vi "labHolo2.vi"() -> ()   [LabVIEW 2022 SP3]
uses:
  <vilib>/Analysis/NI_AALBase.lvlib
panel:
  in  "Mod. func.":string
  in  "SLM calibration":u16(ring) items=["211209_lowFreq", "a20220523", "IDSfirst"]
  in  "Reset reff.":bool
  in  "RefTimeSeries 2":dbl[](array[numeric])=array[4424 elements]
  out "Reff alert":bool
  out "size":i32=378225
  out "Reff ROI":T1={"Global Rectangle"=[2653, 1459, 3268, 2074], "Contours"=[{"Contour Type"=0, "ROI Type"=3, "Points"=[2653, 1459, 3268, 2074]}]}
  in  "RefTimeSeries":dbl[](array[numeric])=array[4424 elements]
  in  "take reff":bool
  out "ROI":T1={"Global Rectangle"=[437, 929, 1461, 1953], "Contours"=[{"Contour Type"=0, "ROI Type"=3, "Points"=[437, 929, 1461, 1953]}]}
  in  "Auto. hist":bool caption="Auto."
  out "ROI size":i32=1048576
  out "mean":dbl=2640.427523612976
  out "mean bar":dbl(slide)=2640.427523612976 scale=0.0..200.0
  in  "Whole/ROI":bool=TRUE
  out "max":i16=4095
  out "Histograph":T2(graph)={"Starting Value"=0.0, "Incremental Value"=1.0002441, "Histogram"=[0, 0, 0, 0, 0, 0, 0, 0, 0, 0, 0, 0, 0, 0, 0, 0, 0, 0, 0, 0, 0, 0, 0, 0, 0, 0, 0, 0, 0, 0, 0, 0, 0, 0, 0, 0, 0, 0, 0, 0, 0, 0, 0, 0, 0, 0, 0, 0, 0, 0, 0, 0, 0, 0, 0, 0, 0, 0, 0, 0, 0, 0, 0, 0, 0, 0, 0, 0, 0, 0, 0, 0, 0, 0, 0, 0, 0, 0, 0, 0, 0, 0, 0, 0, 0, 0, 0, 0, 0, 0, 0, 0, 0, 0, 0, 0, 0, 0, 0, 0, 0, 0, 0, 0, 0, 0, 0, 0, 0, 0, 0, 0, 0, 0, 0, 0, 0, 0, 0, 0, 0, 0, 0, 0, 0, 0, 0, 0, 0, 0, 0, 0, 0, 0, 0, 0, 0, 0, 0, 0, 0, 0, 0, 0, 0, 0, 0, 0, 0, 0, 0, 0, 0, 0, 0, 0, 0, 0, 0, 0, 0, 0, 0, 0, 0, 0, 0, 0, 0, 0, 0, 0, 0, 0, 0, 0, 0, 0, 0, 0, 0, 0, 0, 0, 0, 0, 0, 0, 0, 0, 0, 0, 0, 0, 0, 0, 0, 0, 0, 0, 0, 0, 0, 0, 0, 0, 0, 0, 0, 0, 0, 0, 0, 0, 0, 0, 0, 0, 0, 0, 0, 0, 0, 0, 0, 0, 0, 0, 0, 0, 0, 0, 0, 0, 0, 0, 0, 0, 0, 0, 0, 0, 0, 0, 0, 0, 0, 0, 0, 0, 0, 0, 0, 0, 0, 0, 0, 0, 0, 0, 0, 0, 0, 0, 0, 0, 0, 0, 0, 0, 0, 0, 0, 0, 0, 0, 0, 0, 0, 0, 0, 0, 0, 0, 0, 0, 0, 0, 0, 0, 0, 0, 0, 0, 0, 0, 0, 0, 0, 0, 0, 0, 0, 0, 0, 0, 0, 0, 0, 0, 0, 0, 0, 0, 0, 0, 0, 0, 0, 0, 0, 0, 0, 0, 0, 0, 0, 0, 0, 0, 0, 0, 0, 0, 0, 0, 0, 0, 0, 0, 0, 0, 0, 0, 0, 0, 0, 0, 0, 0, 0, 0, 0, 0, 0, 0, 0, 0, 0, 0, 0, 0, 0, 0, 0, 0, 0, 0, 0, 0, 0, 0, 0, 0, 0, 0, 0, 0, 0, 0, 0, 0, 0, 0, 0, 0, 0, 0, 0, 0, 0, 0, 0, 0, 0, 0, 0, 0, 0, 0, 0, 0, 0, 0, 0, 0, 0, 0, 0, 0, 0, 0, 0, 0, 0, 0, 0, 0, 0, 0, 0, 0, 0, 0, 0, 0, 0, 0, 0, 0, 0, 0, 0, 0, 0, 0, 0, 0, 0, 0, 0, 0, 0, 0, 0, 0, 0, 0, 0, 0, 0, 0, 0, 0, 0, 0, 0, 0, 0, 0, 0, 0, 0, 0, 0, 0, 0, 0, 0, 0, 0, 0, 0, 0, 0, 0, 0, 0, 0, 0, 0, 0, 0, 0, 0, 0, 0, 0, 0, 0, 0, 0, 0, 0, 0, 0, 0, 0, 0, 0, 0, 0, 0, 0, 0, 0, 0, 0, 0, 0, 0, 0, 0, 0, 0, 0, 0, 0, 0, 0, 0, 0, 0, 0, 0, 0, 0, 0, 0, 0, 0, 0, 0, 0, 0, 0, 0, 0, 0, 0, 0, 0, 0, 0, 0, 0, 0, 0, 0, 0, 0, 0, 0, 0, 0, 0, 0, 0, 0, 0, 0, 0, 0, 0, 0, 0, 0, 0, 0, 0, 0, 0, 0, 0, 0, 0, 0, 0, 0, 0, 0, 0, 0, 0, 0, 0, 0, 0, 0, 0, 0, 0, 0, 0, 0, 0, 0, 0, 0, 0, 0, 0, 0, 0, 0, 0, 0, 0, 0, 0, 0, 0, 0, 0, 0, 0, 0, 0, 0, 0, 0, 0, 0, 0, 0, 0, 0, 0, 0, 0, 0, 0, 0, 0, 0, 0, 0, 0, 0, 0, 0, 0, 0, 0, 0, 0, 0, 0, 0, 0, 0, 0, 0, 0, 0, 0, 0, 0, 0, 0, 0, 0, 0, 0, 0, 0, 0, 0, 0, 0, 0, 0, 0, 0, 0, 0, 0, 0, 0, 0, 0, 0, 0, 0, 0, 0, 0, 0, 0, 0, 0, 0, 0, 0, 0, 0, 0, 0, 0, 0, 0, 0, 0, 0, 0, 0, 0, 0, 0, 0, 0, 0, 0, 0, 0, 0, 0, 0, 0, 0, 0, 0, 0, 0, 0, 0, 0, 0, 0, 0, 0, 0, 0, 0, 0, 0, 0, 0, 0, 0, 0, 0, 0, 0, 0, 0, 0, 0, 0, 0, 0, 0, 0, 0, 0, 0, 0, 0, 0, 0, 0, 0, 0, 0, 0, 0, 0, 0, 0, 0, 0, 0, 0, 0, 0, 0, 0, 0, 0, 0, 0, 0, 0, 0, 0, 0, 0, 0, 0, 0, 0, 0, 0, 0, 0, 0, 0, 0, 0, 0, 0, 0, 0, 0, 0, 0, 0, 0, 0, 0, 0, 0, 0, 0, 0, 0, 0, 0, 0, 0, 0, 0, 0, 0, 0, 0, 0, 0, 0, 0, 0, 0, 0, 0, 0, 0, 0, 0, 0, 0, 0, 0, 0, 0, 0, 0, 0, 0, 0, 0, 0, 0, 0, 0, 0, 0, 0, 0, 0, 0, 0, 0, 0, 0, 0, 0, 0, 0, 0, 0, 0, 0, 0, 0, 0, 0, 0, 0, 0, 0, 0, 0, 0, 0, 0, 0, 0, 0, 0, 0, 0, 0, 0, 0, 0, 0, 0, 0, 0, 0, 0, 0, 0, 0, 0, 0, 0, 0, 0, 0, 0, 0, 0, 0, 0, 0, 0, 0, 0, 0, 0, 0, 0, 0, 0, 0, 0, 0, 0, 0, 0, 0, 0, 0, 0, 0, 0, 0, 0, 0, 0, 0, 0, 0, 0, 0, 0, 0, 0, 0, 0, 0, 0, 0, 0, 0, 0, 0, 0, 0, 0, 0, 0, 0, 0, 0, 0, 0, 0, 0, 0, 0, 0, 0, 0, 0, 0, 0, 0, 0, 0, 0, 0, 0, 0, 0, 0, 0, 0, 0, 0, 0, 0, 0, 0, 0, 0, 0, 0, 0, 0, 0, 0, 0, 0, 0, 0, 0, 0, 0, 0, 0, 0, 0, 0, 0, 0, 0, 0, 0, 0, 0, 0, 0, 0, 0, 0, 0, 0, 0, 0, 0, 0, 0, 0, 0, 0, 0, 0, 0, 0, 0, 0, 0, 0, 0, 0, 0, 0, 0, 0, 0, 0, 0, 0, 0, 0, 0, 0, 0, 0, 0, 0, 0, 0, 0, 0, 0, 0, 0, 0, 0, 0, 0, 0, 0, 0, 0, 0, 0, 0, 0, 0, 0, 0, 0, 0, 0, 0, 0, 0, 0, 0, 0, 0, 0, 0, 0, 0, 0, 0, 0, 0, 0, 0, 0, 0, 0, 0, 0, 0, 0, 0, 0, 0, 0, 0, 0, 0, 0, 0, 0, 0, 0, 0, 0, 0, 0, 0, 0, 0, 0, 0, 0, 0, 0, 0, 0, 0, 0, 0, 0, 0, 0, 0, 0, 0, 0, 0, 0, 0, 0, 0, 0, 0, 0, 0, 0, 0, 0, 0, 0, 0, 0, 0, 0, 0, 0, 0, 0, 0, 0, 0, 0, 0, 0, 0, 0, 0, 0, 0, 0, 0, 0, 0, 0, 0, 0, 0, 0, 0, 0, 0, 0, 0, 0, 0, 0, 0, 0, 0, 0, 0, 0, 0, 0, 0, 0, 0, 0, 0, 0, 0, 0, 0, 0, 0, 0, 0, 0, 0, 0, 0, 0, 0, 0, 0, 0, 0, 0, 0, 0, 0, 0, 0, 0, 0, 0, 0, 0, 0, 0, 0, 0, 0, 0, 0, 0, 0, 0, 0, 0, 0, 0, 0, 0, 0, 0, 0, 0, 0, 0, 0, 0, 0, 0, 0, 0, 0, 0, 0, 0, 0, 0, 0, 0, 0, 0, 0, 0, 0, 0, 0, 0, 0, 0, 0, 0, 0, 0, 0, 0, 0, 0, 0, 0, 0, 0, 0, 0, 0, 0, 0, 0, 0, 0, 0, 0, 0, 0, 0, 0, 0, 0, 0, 0, 0, 0, 0, 0, 0, 0, 0, 0, 0, 0, 0, 0, 0, 0, 0, 0, 0, 0, 0, 0, 0, 0, 0, 0, 0, 0, 0, 0, 0, 0, 0, 0, 0, 0, 0, 0, 0, 0, 0, 0, 0, 0, 0, 0, 0, 0, 0, 0, 0, 0, 0, 0, 0, 0, 0, 0, 0, 0, 0, 0, 0, 0, 0, 0, 0, 0, 0, 0, 0, 0, 0, 0, 0, 0, 0, 0, 0, 0, 0, 0, 0, 0, 0, 0, 0, 0, 0, 0, 0, 0, 0, 0, 0, 0, 0, 0, 0, 0, 0, 0, 0, 0, 0, 0, 0, 0, 0, 0, 0, 0, 0, 0, 0, 0, 0, 0, 0, 0, 0, 0, 0, 0, 0, 0, 0, 0, 0, 0, 0, 0, 0, 0, 0, 0, 0, 0, 0, 0, 0, 0, 0, 0, 0, 0, 0, 0, 0, 0, 0, 0, 0, 0, 0, 0, 0, 0, 0, 0, 0, 0, 0, 0, 0, 0, 0, 0, 0, 0, 0, 0, 0, 0, 0, 0, 0, 0, 0, 0, 0, 0, 0, 0, 0, 0, 0, 0, 0, 0, 0, 0, 0, 0, 0, 0, 0, 0, 0, 0, 0, 0, 0, 0, 0, 0, 0, 0, 0, 0, 0, 0, 0, 0, 0, 0, 0, 0, 0, 0, 0, 0, 0, 0, 0, 0, 0, 0, 0, 0, 0, 0, 0, 0, 0, 0, 0, 0, 0, 0, 0, 0, 0, 0, 0, 0, 0, 0, 0, 0, 0, 0, 0, 0, 0, 0, 0, 0, 0, 0, 0, 0, 0, 0, 0, 0, 0, 0, 0, 0, 0, 0, 0, 0, 0, 0, 0, 0, 0, 0, 0, 0, 0, 0, 0, 0, 0, 0, 0, 0, 0, 0, 0, 0, 0, 0, 0, 0, 0, 0, 0, 0, 0, 0, 0, 0, 0, 0, 0, 0, 0, 0, 0, 0, 0, 0, 0, 0, 0, 0, 0, 0, 0, 0, 0, 0, 0, 0, 0, 0, 0, 0, 0, 0, 0, 0, 0, 0, 0, 0, 0, 0, 0, 0, 0, 0, 0, 0, 0, 0, 0, 0, 0, 0, 0, 0, 0, 0, 0, 0, 0, 0, 0, 0, 0, 0, 0, 0, 0, 0, 0, 0, 0, 0, 0, 0, 0, 0, 0, 0, 0, 0, 0, 0, 0, 0, 0, 0, 0, 0, 0, 0, 0, 0, 0, 0, 0, 0, 0, 0, 0, 0, 0, 0, 0, 0, 0, 0, 0, 0, 0, 0, 0, 0, 0, 0, 0, 0, 0, 0, 0, 0, 0, 0, 0, 0, 0, 0, 0, 0, 0, 0, 0, 0, 0, 0, 0, 0, 0, 0, 0, 0, 0, 0, 0, 0, 0, 0, 0, 0, 0, 0, 0, 0, 0, 0, 0, 0, 0, 0, 0, 0, 0, 0, 0, 0, 0, 0, 0, 0, 0, 0, 0, 0, 0, 0, 0, 0, 0, 0, 0, 0, 0, 0, 0, 0, 0, 0, 0, 0, 0, 0, 0, 0, 0, 0, 0, 0, 0, 0, 0, 0, 0, 0, 0, 0, 0, 0, 0, 0, 0, 0, 0, 0, 0, 0, 0, 0, 0, 0, 0, 0, 0, 0, 0, 0, 0, 0, 0, 0, 0, 0, 0, 0, 0, 0, 0, 0, 0, 0, 0, 0, 0, 0, 0, 0, 0, 0, 0, 0, 0, 0, 0, 0, 0, 0, 0, 0, 0, 0, 0, 0, 0, 0, 0, 0, 0, 0, 0, 0, 0, 0, 0, 0, 0, 0, 0, 0, 0, 0, 0, 0, 0, 0, 0, 0, 0, 0, 0, 0, 0, 0, 0, 0, 0, 0, 0, 0, 0, 0, 0, 0, 0, 0, 0, 0, 0, 0, 0, 0, 0, 0, 0, 0, 0, 0, 0, 0, 0, 0, 0, 0, 0, 0, 0, 0, 0, 0, 0, 0, 0, 0, 0, 0, 0, 0, 0, 0, 0, 0, 0, 0, 0, 0, 0, 0, 0, 0, 0, 0, 0, 0, 0, 0, 0, 0, 0, 0, 0, 0, 0, 0, 0, 0, 0, 0, 0, 0, 0, 0, 0, 0, 0, 0, 0, 0, 0, 0, 0, 0, 0, 0, 0, 0, 0, 0, 0, 0, 0, 0, 0, 0, 0, 0, 0, 0, 0, 0, 0, 0, 0, 0, 0, 0, 0, 0, 0, 0, 0, 0, 0, 0, 0, 0, 0, 0, 0, 0, 0, 0, 0, 0, 0, 0, 0, 0, 0, 0, 0, 0, 0, 0, 0, 0, 0, 0, 0, 0, 0, 0, 0, 0, 0, 0, 0, 0, 0, 0, 0, 0, 0, 0, 0, 0, 0, 0, 0, 0, 0, 0, 0, 0, 0, 0, 0, 0, 0, 0, 0, 0, 0, 0, 0, 0, 0, 0, 0, 0, 0, 0, 0, 0, 0, 0, 0, 0, 0, 0, 0, 0, 0, 0, 0, 0, 0, 0, 0, 0, 0, 0, 0, 0, 0, 0, 0, 0, 0, 0, 0, 0, 0, 0, 0, 0, 0, 0, 0, 0, 0, 0, 0, 0, 0, 0, 0, 0, 0, 0, 0, 0, 0, 0, 0, 0, 0, 0, 0, 0, 0, 0, 0, 0, 0, 0, 0, 0, 0, 0, 0, 0, 0, 0, 0, 0, 0, 0, 0, 0, 0, 0, 0, 0, 0, 0, 0, 0, 0, 0, 0, 0, 0, 0, 0, 0, 0, 0, 0, 0, 0, 0, 0, 0, 0, 0, 0, 0, 0, 0, 0, 0, 0, 0, 0, 0, 0, 0, 0, 0, 0, 0, 0, 0, 0, 0, 0, 0, 0, 0, 0, 0, 0, 0, 0, 0, 0, 0, 0, 0, 0, 0, 0, 0, 0, 0, 0, 0, 0, 0, 0, 0, 0, 0, 0, 0, 0, 0, 0, 0, 0, 0, 0, 0, 0, 0, 0, 0, 0, 0, 0, 0, 0, 0, 0, 0, 0, 0, 0, 0, 0, 0, 0, 0, 0, 0, 0, 0, 0, 0, 0, 0, 0, 0, 0, 0, 0, 0, 0, 0, 0, 0, 0, 0, 0, 0, 0, 0, 0, 0, 0, 0, 0, 0, 0, 0, 0, 1, 1, 1, 0, 0, 1, 0, 1, 1, 1, 0, 3, 2, 2, 1, 3, 0, 1, 3, 1, 1, 1, 4, 1, 4, 2, 3, 5, 6, 1, 4, 5, 5, 5, 4, 6, 1, 3, 5, 6, 4, 4, 10, 7, 6, 10, 12, 10, 10, 14, 17, 7, 19, 19, 16, 14, 16, 14, 30, 22, 26, 33, 30, 27, 43, 34, 52, 34, 41, 41, 39, 39, 46, 59, 56, 57, 62, 62, 78, 61, 67, 70, 87, 72, 81, 78, 110, 96, 92, 129, 120, 133, 128, 122, 160, 139, 167, 147, 170, 165, 189, 191, 196, 233, 217, 218, 232, 249, 252, 278, 271, 270, 295, 307, 360, 311, 348, 338, 375, 377, 388, 376, 421, 443, 443, 436, 462, 520, 517, 558, 604, 575, 584, 622, 662, 711, 666, 732, 747, 741, 812, 804, 797, 839, 839, 875, 848, 986, 977, 981, 946, 1009, 1094, 1088, 1095, 1100, 1154, 1186, 1234, 1270, 1228, 1266, 1333, 1337, 1349, 1444, 1418, 1489, 1508, 1532, 1606, 1526, 1650, 1589, 1647, 1705, 1742, 1730, 1788, 1825, 1847, 1852, 1889, 1974, 1898, 1933, 2035, 2073, 2118, 2106, 2143, 2225, 2197, 2147, 2281, 2381, 2372, 2326, 2423, 2349, 2326, 2463, 2436, 2555, 2545, 2437, 2626, 2580, 2594, 2658, 2697, 2728, 2720, 2712, 2674, 2845, 2701, 2720, 2851, 2864, 2959, 2873, 2957, 2922, 2913, 2950, 3091, 2945, 2974, 2955, 3011, 3050, 3132, 3059, 3105, 3081, 3040, 3219, 3171, 3107, 3191, 3160, 3078, 3201, 3173, 3152, 3136, 3301, 3251, 3254, 3355, 3257, 3247, 3179, 3175, 3207, 3183, 3338, 3322, 3418, 3293, 3159, 3334, 3349, 3401, 3334, 3449, 3403, 3253, 3249, 3353, 3281, 3382, 3411, 3345, 3317, 3299, 3254, 3346, 3342, 3353, 3361, 3274, 3357, 3329, 3316, 3298, 3251, 3273, 3229, 3209, 3295, 3252, 3293, 3361, 3317, 3258, 3311, 3345, 3317, 3270, 3263, 3261, 3219, 3393, 3311, 3273, 3299, 3325, 3323, 3237, 3304, 3349, 3390, 3230, 3284, 3321, 3277, 3296, 3227, 3344, 3322, 3218, 3297, 3322, 3269, 3284, 3304, 3343, 3415, 3328, 3360, 3383, 3311, 3384, 3402, 3244, 3399, 3273, 3256, 3404, 3336, 3392, 3368, 3411, 3419, 3326, 3342, 3464, 3470, 3273, 3343, 3342, 3268, 3436, 3407, 3437, 3405, 3425, 3425, 3428, 3310, 3508, 3385, 3258, 3413, 3348, 3374, 3409, 3341, 3344, 3404, 3459, 3451, 3383, 3392, 3367, 3533, 3359, 3574, 3386, 3436, 3385, 3397, 3345, 3448, 3409, 3462, 3418, 3486, 3312, 3401, 3533, 3445, 3394, 3429, 3366, 3473, 3421, 3389, 3368, 3424, 3485, 3388, 3247, 3405, 3358, 3438, 3188, 3324, 3359, 3281, 3258, 3212, 3207, 3310, 3208, 3162, 3238, 3200, 3161, 3088, 3168, 3130, 3175, 3159, 3044, 3031, 3019, 3006, 2940, 3030, 3076, 3024, 2976, 2788, 2872, 2868, 2797, 2852, 2830, 2890, 2752, 2688, 2758, 2676, 2590, 2590, 2669, 2616, 2600, 2560, 2532, 2417, 2428, 2385, 2481, 2456, 2305, 2295, 2295, 2207, 2270, 2275, 2238, 2135, 1992, 2114, 2097, 2022, 2006, 1946, 1929, 1882, 1880, 1831, 1800, 1804, 1743, 1739, 1675, 1696, 1573, 1680, 1563, 1614, 1401, 1500, 1501, 1440, 1376, 1371, 1386, 1314, 1302, 1275, 1273, 1246, 1148, 1240, 1151, 1161, 1092, 1082, 1041, 1028, 1010, 1003, 913, 947, 883, 875, 900, 843, 804, 820, 735, 716, 730, 747, 687, 694, 660, 666, 593, 611, 616, 571, 563, 570, 518, 540, 509, 454, 486, 470, 416, 408, 391, 404, 382, 390, 367, 348, 308, 306, 303, 291, 298, 278, 278, 259, 249, 235, 250, 225, 206, 206, 206, 186, 197, 173, 199, 191, 157, 154, 159, 128, 117, 135, 136, 113, 134, 122, 114, 94, 105, 89, 96, 108, 100, 83, 79, 74, 82, 85, 61, 62, 56, 74, 69, 60, 64, 55, 53, 47, 51, 49, 43, 39, 39, 32, 36, 36, 46, 36, 35, 25, 32, 25, 33, 25, 26, 27, 28, 21, 19, 18, 18, 25, 21, 33, 22, 17, 15, 17, 19, 20, 18, 13, 25, 16, 19, 17, 15, 12, 15, 10, 9, 11, 19, 10, 12, 8, 15, 14, 9, 9, 11, 14, 13, 11, 12, 9, 11, 7, 9, 5, 6, 6, 9, 16, 7, 8, 13, 5, 6, 11, 9, 5, 8, 6, 8, 5, 7, 8, 3, 8, 4, 8, 3, 4, 6, 7, 4, 4, 6, 5, 2, 5, 6, 6, 10, 2, 5, 7, 6, 2, 3, 3, 7, 5, 6, 3, 7, 5, 4, 7, 3, 2, 9, 1, 9, 3, 2, 6, 1, 3, 1, 6, 2, 2, 1, 5, 1, 2, 2, 2, 4, 1, 3, 2, 5, 1, 2, 2, 1, 1, 4, 1, 2, 6, 2, 0, 4, 1, 1, 4, 2, 1, 1, 1, 3, 1, 3, 2, 2, 3, 1, 1, 4, 3, 0, 0, 5, 0, 1, 3, 0, 1, 1, 3, 3, 4, 2, 2, 1, 2, 2, 2, 4, 0, 1, 3, 1, 3, 0, 1, 0, 1, 3, 1, 4, 2, 0, 1, 3, 1, 0, 3, 3, 1, 2, 4, 2, 2, 2, 2, 0, 1, 2, 2, 2, 1, 6, 0, 0, 1, 0, 3, 2, 1, 3, 1, 3, 2, 2, 3, 3, 2, 2, 2, 2, 1, 1, 0, 1, 2, 1, 1, 1, 1, 2, 3, 1, 3, 0, 1, 2, 2, 2, 3, 2, 1, 1, 1, 0, 1, 2, 2, 3, 0, 5, 0, 2, 1, 3, 1, 0, 1, 2, 2, 1, 1, 3, 3, 4, 2, 1, 0, 4, 0, 0, 0, 0, 4, 1, 1, 0, 0, 1, 3, 2, 1, 3, 4, 0, 3, 1, 3, 5, 0, 1, 2, 2, 1, 1, 2, 1, 4, 0, 1, 1, 3, 0, 0, 1, 0, 2, 1, 1, 1, 2, 1, 1, 2, 2, 5, 2, 0, 0, 2, 0, 1, 1, 2, 0, 0, 2, 1, 1, 2, 2, 3, 1, 0, 2, 1, 2, 2, 2, 2, 4, 0, 1, 4, 0, 1, 1, 3, 0, 2, 4, 1, 0, 2, 1, 3, 2, 0, 3, 3, 0, 2, 1, 0, 0, 1, 0, 1, 0, 2, 1, 2, 1, 3, 1, 1, 1, 0, 3, 2, 1, 0, 1, 2, 0, 1, 2, 0, 2, 2, 2, 1, 0, 0, 0, 2, 1, 1, 4, 2, 1, 1, 0, 0, 2, 0, 0, 2, 2, 2, 0, 1, 2, 1, 0, 1, 1, 1, 2, 1, 0, 1, 0, 2, 2, 2, 2, 0, 0, 0, 0, 1, 3, 1, 1, 0, 2, 1, 1, 2, 0, 1, 2, 3, 1, 0, 0, 3, 0, 1, 0, 2, 0, 1, 0, 3, 0, 0, 0, 2, 1, 3, 2, 3, 2, 1, 2, 3, 0, 3, 0, 0, 1, 2, 1, 0, 2, 2, 2, 0, 1, 0, 2, 3, 0, 1, 2, 1, 2, 1, 0, 1, 1, 0, 0, 2, 3, 0, 1, 1, 1, 1, 1, 0, 1, 2, 3, 0, 3, 1, 3, 0, 1, 1, 1, 1, 0, 0, 1, 0, 0, 0, 1, 2, 0, 0, 0, 1, 0, 0, 1, 1, 0, 2, 1, 2, 2, 2, 0, 0, 1, 1, 3, 0, 1, 2, 0, 1, 1, 0, 2, 1, 1, 2, 1, 0, 2, 0, 0, 0, 3, 0, 1, 2, 1, 1, 1, 1, 2, 2, 0, 1, 1, 0, 3, 3, 1, 0, 0, 0, 0, 1, 0, 1, 1, 2, 2, 0, 0, 1, 1, 2, 3, 0, 2, 0, 1, 0, 0, 2, 2, 0, 1, 0, 0, 2, 2, 1, 2, 0, 0, 0, 0, 0, 2, 0, 3, 3, 0, 0, 2, 2, 1, 1, 0, 1, 0, 0, 0, 2, 1, 1, 1, 2, 1, 4, 0, 1, 0, 2, 0, 0, 1, 2, 0, 1, 0, 0, 0, 0, 1, 0, 0, 1, 1, 3, 1, 1, 2, 0, 1, 0, 2, 2, 1, 0, 1, 0, 1, 0, 0, 1, 2, 0, 2, 0, 1, 3, 2, 1, 2, 4, 1, 0, 1, 3, 1, 1, 4, 1, 0, 1, 0, 0, 1, 1, 1, 2, 3, 0, 1, 2, 3, 0, 1, 0, 2, 1, 0, 2, 2, 0, 2, 1, 0, 1, 0, 0, 1, 1, 2, 1, 0, 2, 2, 1, 0, 0, 2, 0, 1, 0, 0, 0, 3, 0, 0, 1, 1, 0, 0, 0, 2, 0, 0, 0, 1, 2, 1, 2, 1, 1, 1, 1, 0, 0, 2, 1, 0, 0, 2, 2, 0, 2, 2, 2, 1, 0, 0, 1, 1, 1, 2, 0, 0, 2, 1, 1, 1, 0, 1, 1, 0, 1, 0, 1, 0, 0, 2, 2, 0, 1, 0, 0, 1, 0, 0, 1, 1, 2, 1, 0, 0, 1, 1, 1, 0, 2, 0, 1, 0, 2, 0, 0, 0, 0, 1, 0, 2, 0, 3, 1, 0, 1, 0, 0, 0, 0, 0, 1, 2, 0, 1, 0, 1, 2, 2, 1, 1, 2, 1, 1, 0, 0, 0, 0, 0, 1, 1, 2, 1, 1, 1, 0, 0, 1, 0, 0, 1, 0, 0, 0, 1, 2, 0, 1, 0, 0, 1, 1, 0, 0, 1, 1, 3, 1, 0, 0, 0, 1, 0, 3, 0, 0, 1, 0, 1, 0, 1, 1, 1, 0, 1, 0, 1, 1, 1, 1, 0, 1, 0, 1, 1, 0, 1, 2, 0, 1, 1, 1, 0, 0, 1, 1, 0, 1, 2, 1, 1, 1, 1, 0, 1, 0, 1, 0, 1, 3, 0, 0, 0, 1, 1, 0, 0, 0, 0, 0, 0, 0, 0, 0, 0, 1, 1, 1, 0, 0, 1, 0, 1, 1, 0, 0, 0, 0, 1, 1, 2, 0, 3, 1, 0, 0, 0, 0, 0, 0, 2, 1, 0, 1, 0, 3, 2, 0, 0, 1, 0, 1, 1, 0, 0, 0, 1, 1, 0, 2, 1, 0, 1, 0, 1, 0, 0, 0, 1, 0, 0, 1, 0, 0, 1, 2, 2, 1, 0, 0, 1, 2, 1, 1, 0, 0, 0, 0, 0, 0, 1, 0, 0, 1, 2, 0, 0, 2, 1, 0, 1, 0, 1, 1, 0, 0, 0, 0, 2, 0, 0, 0, 1, 1, 0, 1, 1, 1, 0, 2, 0, 1, 0, 0, 1, 0, 0, 0, 1, 0, 0, 0, 0, 0, 2, 0, 0, 1, 0, 0, 0, 0, 1, 1, 0, 2, 0, 0, 0, 0, 0, 0, 1, 0, 0, 1, 0, 0, 0, 0, 0, 0, 1, 0, 0, 1, 1, 0, 0, 0, 0, 0, 0, 0, 0, 0, 0, 1, 0, 0, 0, 0, 0, 0, 0, 0, 0, 0, 0, 1, 0, 0, 1, 0, 0, 0, 0, 0, 0, 0, 0, 0, 1, 0, 0, 0, 1, 0, 0, 0, 0, 0, 0, 0, 1, 1, 1, 1, 0, 0, 0, 0, 0, 0, 1, 0, 1, 0, 0, 0, 0, 0, 1, 0, 0, 2, 1, 0, 0, 0, 1, 0, 0, 0, 0, 295, 0]}
  out "# Sat. Pixels":sgl(slide)=295.0 scale=0.0..10.0
  in  "beam_name":string="topoCharge9"
  out "defaultPath":string="topoCharge9_m+1_pAzi_aLev_z2.png"
  in  "Analyzer":string(combo)="Lev"
  in  "Polarizer":string="Azi"
  in  "suffix":string="z2"
  in  "Save":bool
  out "FPSs":dbl[](array[numeric])=[3.9798457395711155]
  out "exposures":dbl[](array[numeric])=[150.96276094276095]
  in  "Camera ID":u16(ring) caption="Camera" items=["NotFound"]
  out "Real FPS":dbl=4.032258064516129 max=26.76659528907923 format="%#.2g"
  out "py error":errorcluster
  out "CCD Image":T3(plugin-control)
  out "image_size":cluster{"x":i32, "y":i32}={"x"=3816, "y"=2160}
  out "camera attr":T4={"x"=3816, "y"=2160, "FPS"=3.9798457395711155, "Exposure"=150.96276094276095}
  out "1_posCluster":T5={"1_Xoffset"=1329.0, "1_Yoffset"=-67.0, "1_Xgros"=0.04792332268370547, "1_Ygros"=-0.08130081300812986, "1_Xfine"=-1.2939297124600642, "1_Yfine"=0.18218623481781382}
  out "path editor log":errorcluster caption="error out"
  out "SLM1 cluster":T6={"1_Radio"=enum."Radio Selection 5", "1_Trans"=100.0, "1_Phase"=0.0, "1_HoloCode"="dfhdfgh", "1_Semi"=TRUE, "1_Active"=0, "1_ModType"="_complex", "1_Flip"="no flip", "HoloNum"=87.0, "paramStr"="s", "paramVal"=-1, "paramAux"="m+1"}
  in  "paramStr":string="s" caption="Parameters"
  in  "paramVal":i64=-1
  in  "HoloNum":dbl=87.0 caption="Holo:"
  out "1_HoloName":string
  in  "paramAux":string="m+1" caption="String 5"
  in  "SLMs Main":enum32{"SLM 1", "SLM 2"}(tab)
  in  "1_SLMtab":T7(tab) caption="SLM 1:"
  out "CGH_1":T3(plugin-control)
  in  "1_Ygros":dbl(slide)=-0.08130081300812986 scale=-5.0..5.0
  in  "1_Xgros":dbl(slide)=0.04792332268370547 caption="X Possition:" scale=-5.0..5.0
  in  "1_Xfine":dbl(slide)=-1.2939297124600642 caption="fine:" scale=-5.0..5.0
  in  "1_Yfine":dbl(slide)=0.18218623481781382 caption="Fine:" scale=-5.0..5.0
  in  "1_Xoffset":dbl=1329.0
  in  "1_Yoffset":dbl=-67.0 caption="Yoffset"
  out "1_Xpos":dbl=1324.926517571885
  out "1_Ypos":dbl=-63.84589052368258
  in  "1_HoloCode":string="dfhdfgh" caption="Hologram code"
  out "SLM1 path":path=path "C:/Users/dmaluenda/OneDrive - Universitat de Barcelona/Research/pyHolo/Holograms/87_s-1_m+1_complex.png"
  out "1_Int":dbl=1.0
  in  "1_Radio":T8(radio)=enum."Radio Selection 5"
  in  "1_Semi":bool=TRUE caption="Boolean"
  in  "1_ModType":string(combo)="_complex" caption="Modulation curve"
  out "1_PhRad":dbl
  out "1_Tgl":dbl=255.0 caption="[0 255]"
  out "1_PhDeg":dbl
  in  "1_Phase":dbl(slide) caption="Phase:" scale=0.0..360.0
  out "1_T%":dbl=100.0
  in  "1_Trans":dbl(slide)=100.0 caption="Trans.:\n(Amp.)" scale=0.0..100.0
  out "SLM1 monitor":T3(plugin-control)
  in  "1_Flip":string(combo)="no flip" caption="Flip"
  out "Beam1":T3(plugin-control)
  in  "1_Active":u16(ring) items=["ON", "OFF", "edit"]
  in  "2_SLMtab":enum32{"Viewer & Positioner", "Hologram Loader"}(tab)=enum."Hologram Loader" caption="SLM 2:"
  out "CGH_2":T3(plugin-control)
  in  "2_Ygros":dbl(slide)=-0.5284552845528454 scale=-5.0..5.0
  in  "2_Xgros":dbl(slide)=2.7955271565495208 caption="X Possition:" scale=-5.0..5.0
  in  "2_Xfine":dbl(slide)=-0.20766773162939334 caption="fine:" scale=-5.0..5.0
  in  "2_Yfine":dbl(slide)=-0.5060728744939267 caption="Fine:" scale=-5.0..5.0
  out "String 2":string
  in  "2_Xoffset":dbl=1280.0
  in  "2_Yoffset":dbl caption="Yoffset"
  out "2_Xpos":dbl=1418.7380191693292
  out "2_Ypos":dbl=28.953128600111903
  in  "2_HoloCode":string caption="Hologram code"
  out "SLM2 path":path=path "C:/Users/dmaluenda/OneDrive - Universitat de Barcelona/Research/pyHolo/Holograms/87_s-1_m+1_complex.png"
  out "2_Int":dbl=100.0
  in  "2_Radio":T8(radio)=enum."Radio Selection 2"
  in  "2_Semi":bool caption="Boolean"
  in  "2_ModType":string(combo)="_complex" caption="Modulation curve"
  out "2_PhRad":dbl
  out "2_Tgl":dbl caption="[0 255]"
  out "2_PhDeg":dbl
  in  "2_Phase":dbl(slide) caption="Phase:" scale=0.0..360.0
  out "2_T%":dbl=100.0
  in  "2_Trans":dbl(slide)=100.0 caption="Trans.:\n(Amp.)" scale=0.0..100.0
  out "SLM2 monitor":T3(plugin-control)
  in  "2_Active":bool=TRUE
  in  "2_Flip":string(combo)="no flip" caption="Flip"
  out "available\ncameras":cluster{string[], string[]}={["U3-38JxXLE-M"], ["4104527767"]}
  in  "FPS":dbl=3.9798457395711155 format="%#_4g"
  in  "Exposure (ms)":dbl=150.96276094276095 format="%#.3g"
  in  "bit depth":enum16{"16bits", "14bits", "12bits", "8bits"}(ring)=enum."12bits"
  in  "Parada Total":bool
  out "path":path=path "C:/Users/dmaluenda/OneDrive - Universitat de Barcelona/Research/pyHolo/gui"
  out "Chart TimeSeries":dbl[][](graph) caption="Reff. TimeSeries"
  # "Positions:"
  # "X:"
  # "Y:"
  # "Y position:"
  # "Arbitrary value settings:"
  # "For gray levels ->"
  # "%"
  # "Amp"
  # "Int."
  # "º"
  # "\\pi rad"
  # "Positions:"
  # "X:"
  # "Y:"
  # "Y position:"
  # "Arbitrary value settings:"
  # "For gray levels ->"
  # "%"
  # "Amp"
  # "Int."
  # "º"
  # "\\pi rad"
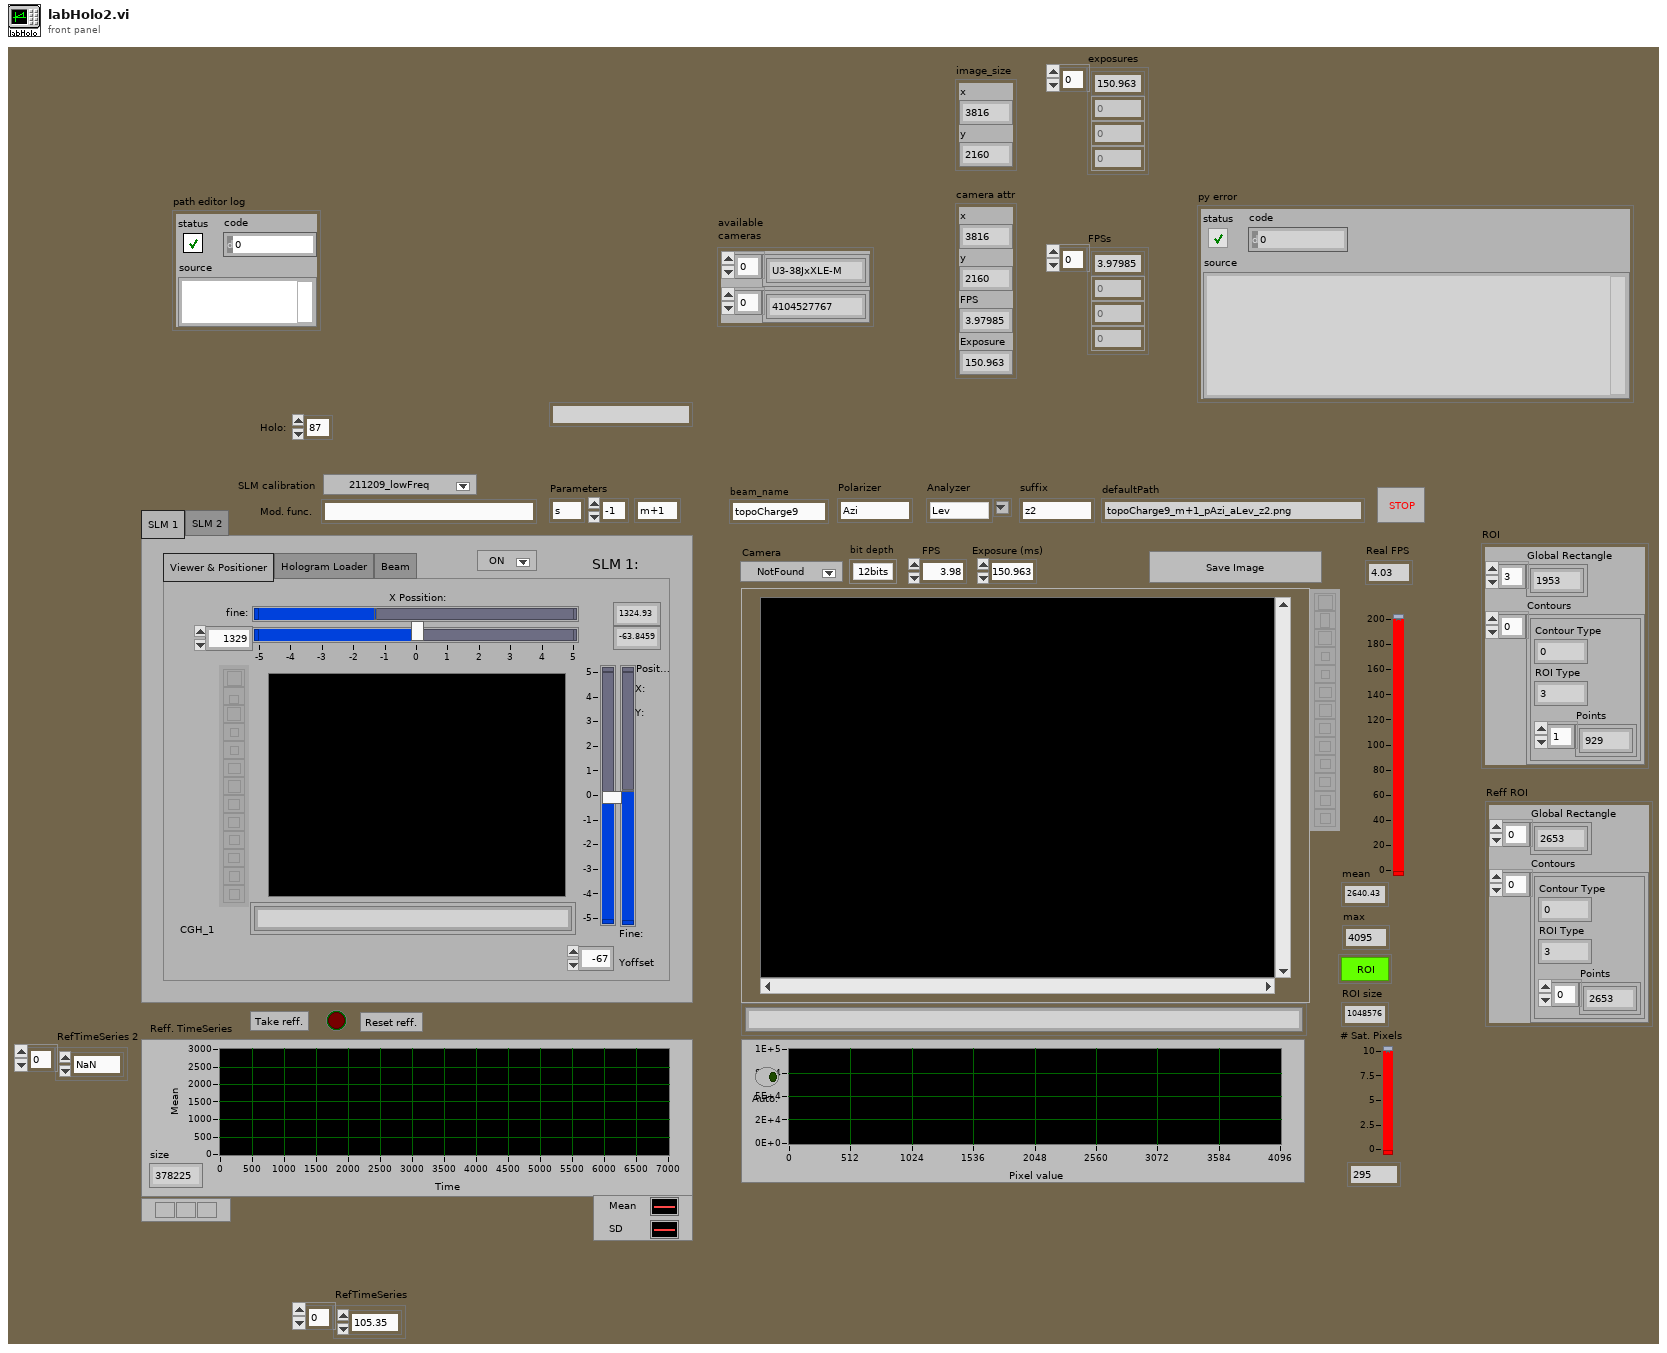
[diagram p1: front panel]
types:
  T1 = cluster{"Global Rectangle":i32[], "Contours":cluster{"Contour Type":u32, "ROI Type":u32, "Points":i32[]}[]}
  T2 = cluster{"Starting Value":sgl, "Incremental Value":sgl, "Histogram":u32[]}
  T3 = typedef "IMAQ Image.ctl" = refnum<image>
  T4 = cluster{"x":i32, "y":i32, "FPS":dbl, "Exposure":dbl}
  T5 = cluster{"1_Xoffset":dbl, "1_Yoffset":dbl, "1_Xgros":dbl, "1_Ygros":dbl, "1_Xfine":dbl, "1_Yfine":dbl}
  T6 = cluster{"1_Radio":enum32{"Radio Selection 1", "Radio Selection 2", "Radio Selection 3", "Radio Selection 4", "Radio Selection 5", "Radio Selection 6", "Radio Selection 7", "Radio Selection 8"}, "1_Trans":dbl, "1_Phase":dbl, "1_HoloCode":string, "1_Semi":bool, "1_Active":u16, "1_ModType":string, "1_Flip":string, "HoloNum":dbl, "paramStr":string, "paramVal":i64, "paramAux":string}
  T7 = enum32{"Viewer & Positioner", "Hologram Loader", "Beam"}
  T8 = enum32{"Radio Selection 1", "Radio Selection 2", "Radio Selection 3", "Radio Selection 4", "Radio Selection 5", "Radio Selection 6", "Radio Selection 7", "Radio Selection 8"}
  T9 = enum8{"Enabled", "Disabled", "Disabled and Grayed Out"}
  T10 = typedef "Image Type" = u32
  T11 = cluster{"2_Xoffset":dbl, "2_Yoffset":dbl, "2_Xgros":dbl, "2_Ygros":dbl, "2_Xfine":dbl, "2_Yfine":dbl}
  T12 = cluster{"mean (ROI)":dbl, "max (ROI)":i16, "max_counts":dbl, "image_size":i32, "# Sat. Pixels":sgl, "# in percentile":dbl}
  T13 = cluster{"1_Radio":enum32{"Radio Selection 1", "Radio Selection 2", "Radio Selection 3", "Radio Selection 4", "Radio Selection 5", "Radio Selection 6", "Radio Selection 7", "Radio Selection 8"}, "1_Trans":dbl, "1_Phase":dbl, "HoloCode 1":string, "1_Semi":bool, "1_Active":u16, "1_ModType":string, "1_Flip":string, "HoloNum":dbl, "ParamStr":string, "ParamVal":dbl, "ParamAux":string}
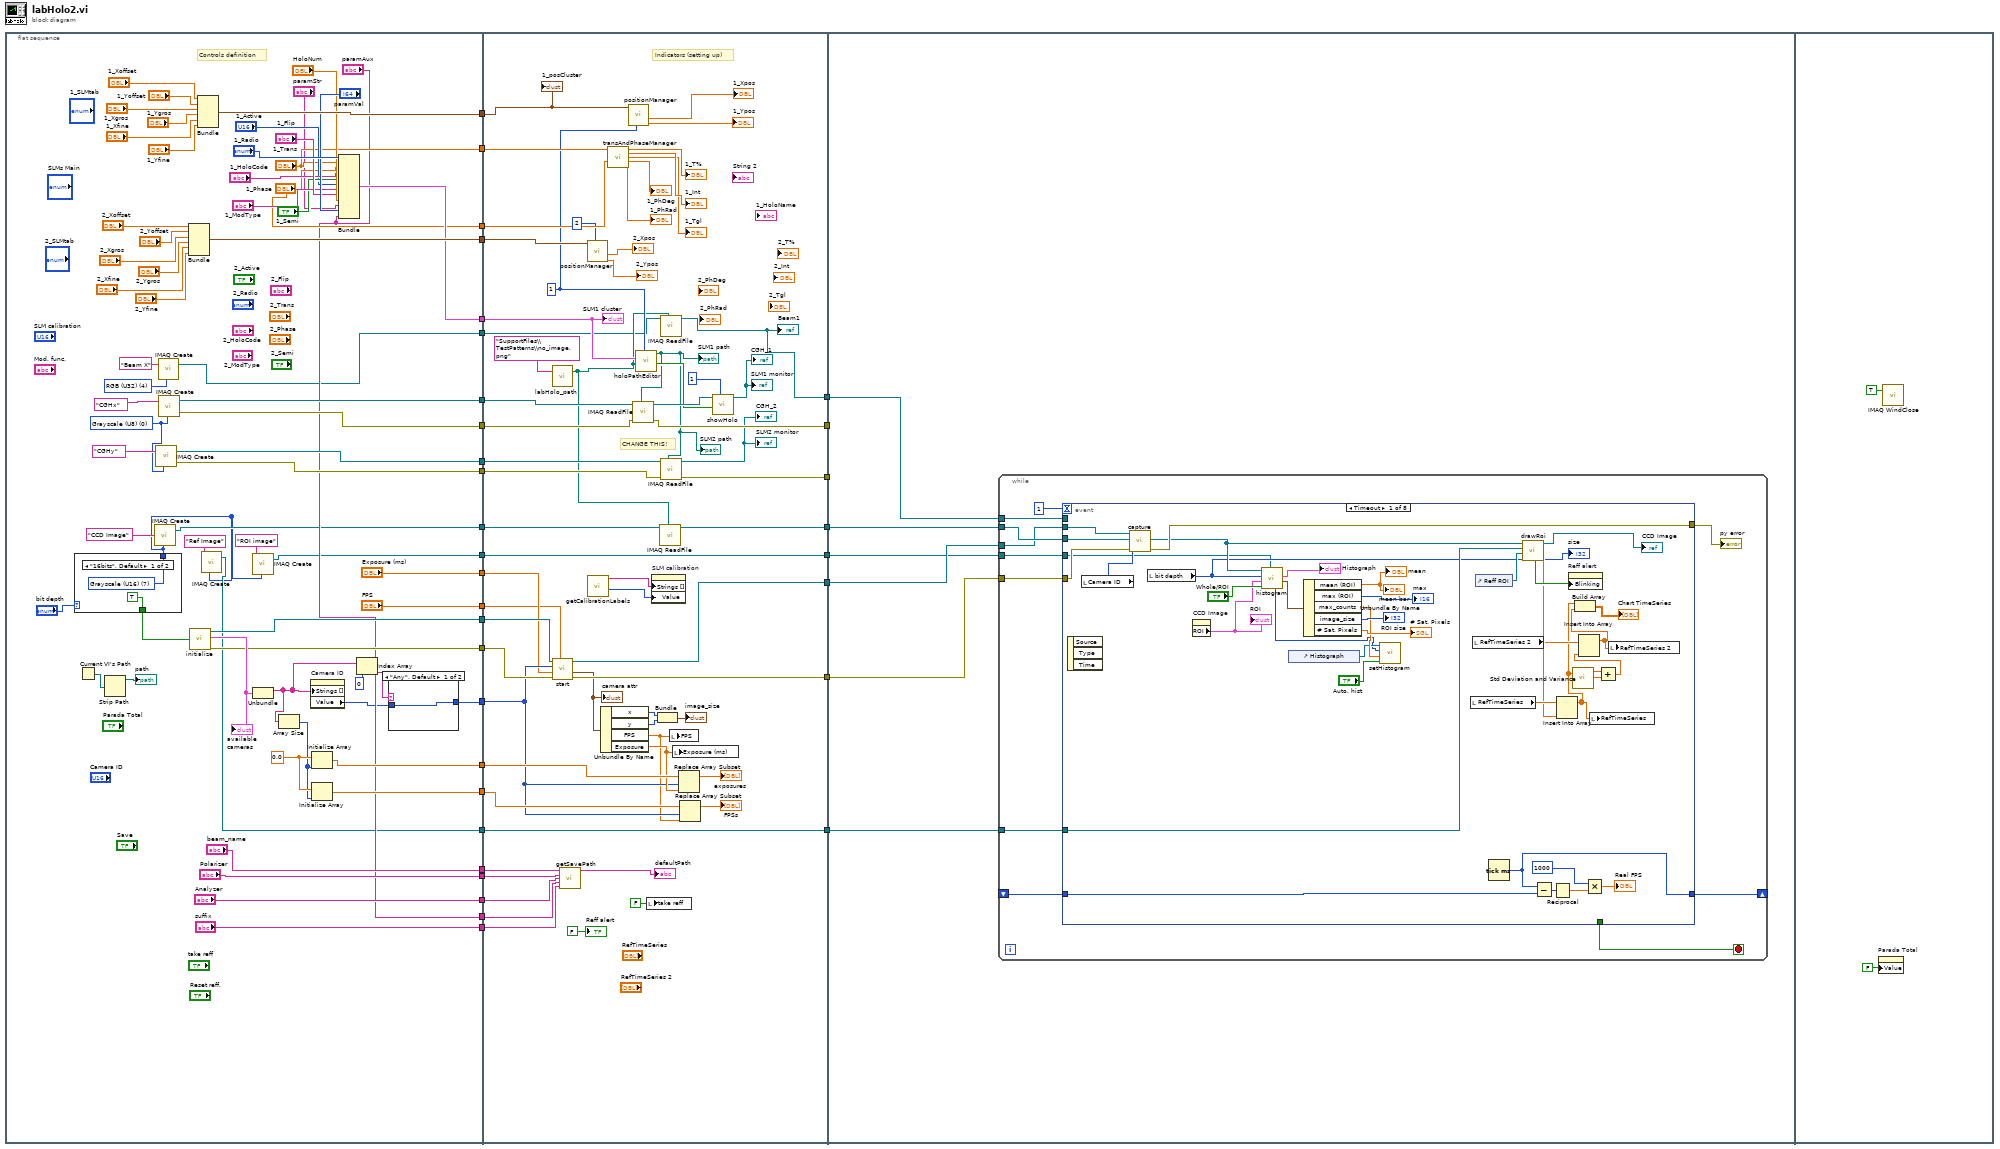
[diagram p0: block diagram]
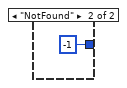
[diagram p2: hidden frame]
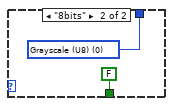
[diagram p3: hidden frame]
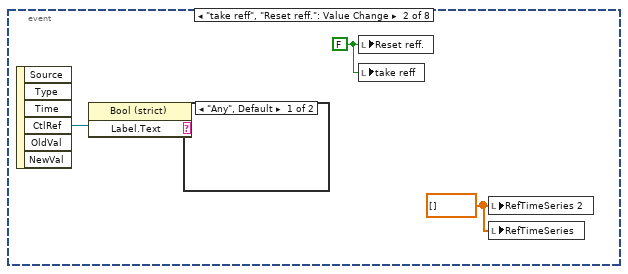
[diagram p4: hidden frame]
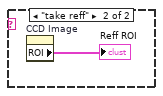
[diagram p5: hidden frame]
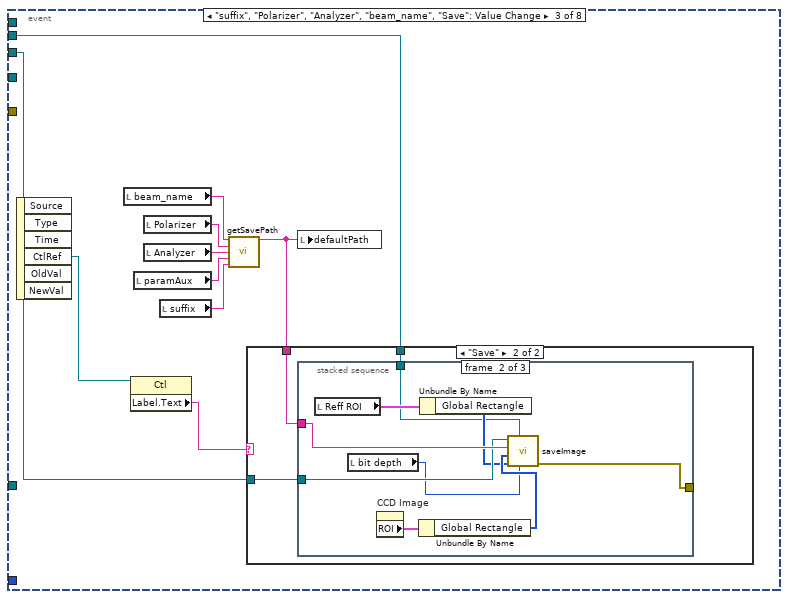
[diagram p6: hidden frame]
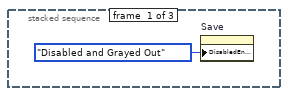
[diagram p8: hidden frame]
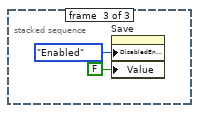
[diagram p9: hidden frame]
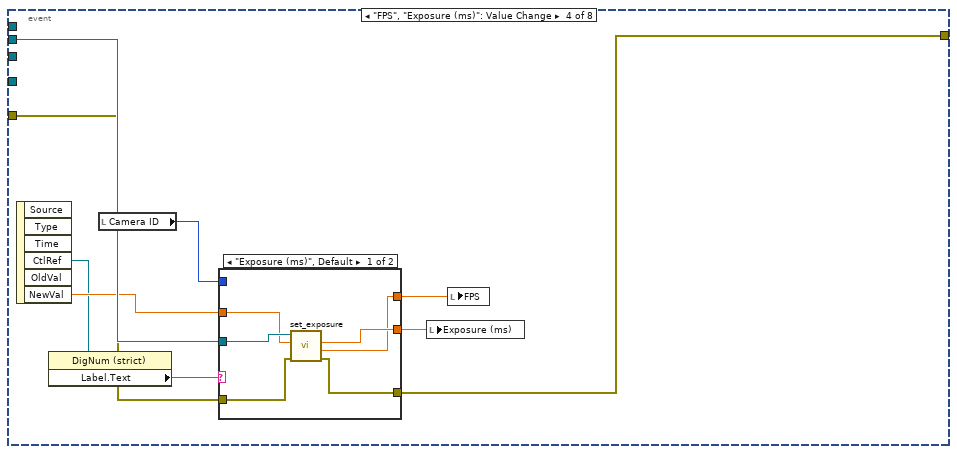
[diagram p10: hidden frame]
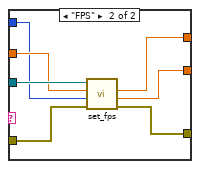
[diagram p11: hidden frame]
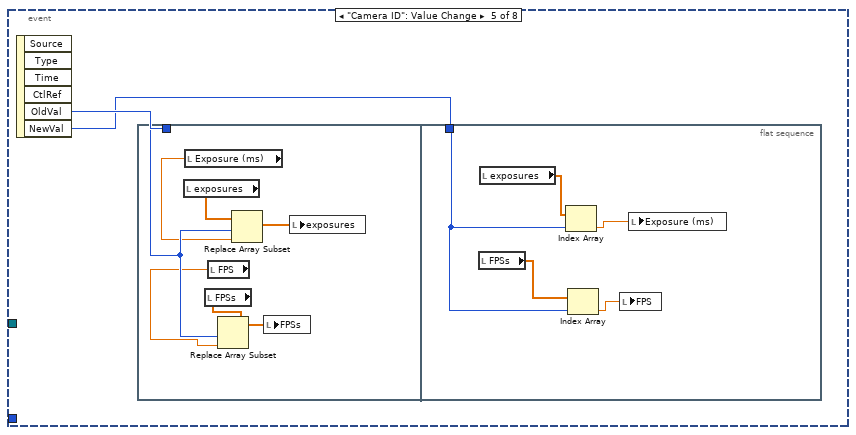
[diagram p12: hidden frame]
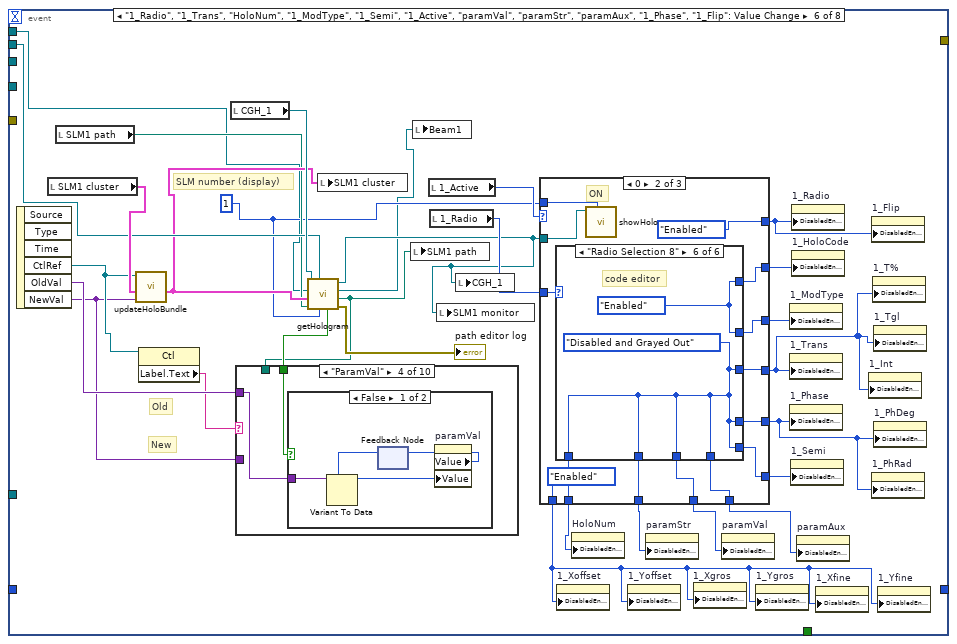
[diagram p13: hidden frame]
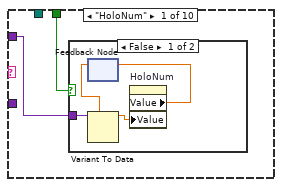
[diagram p14: hidden frame]
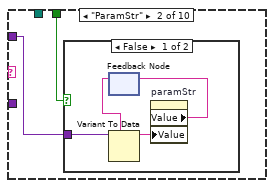
[diagram p16: hidden frame]
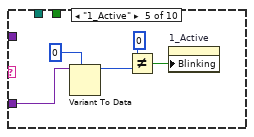
[diagram p20: hidden frame]
diagram:
  n1 = flat-sequence {
    tunnel: [w97] -> w33
    tunnel: [w96] -> w32
    tunnel: [w95] -> w31
    tunnel: [w94] -> w30
    tunnel: [w84] -> w29
    tunnel: [w77] -> w23
    tunnel: [w68] -> w22
    tunnel: ["1_Trans"] -> w21
    tunnel: ["1_Phase"] -> w20
    tunnel: [w64] -> w19
    tunnel: [w42] -> w18
    tunnel: [w63] -> w17
    tunnel: [w62] -> w16
    tunnel: [w59] -> w15
    tunnel: ["Exposure (ms)"] -> w14
    tunnel: ["FPS"] -> w13
    tunnel: ["beam_name"] -> w12
    tunnel: ["Polarizer"] -> w11
    tunnel: ["Analyzer"] -> w10
    tunnel: ["suffix"] -> w9
    tunnel: ["paramAux"] -> w8
    tunnel: [w48] -> w7
    tunnel: [w46] -> w5
    tunnel: [w43] -> w3
    tunnel: [w34] -> w2
    tunnel: w33 -> [w165]
    tunnel: w32 -> [w162]
    tunnel: w31 -> [w161]
    tunnel: w30 -> [w164]
    tunnel: w29 -> [w168]
    tunnel: [w163] -> w28
    tunnel: [w117] -> w27
    tunnel: [w134] -> w26
    tunnel: [w136] -> w25
    tunnel: [w160] -> w24
    tunnel: w23 -> [w159]
    tunnel: w22 -> [w149]
    tunnel: w21 -> [w151]
    tunnel: w20 -> [w150]
    tunnel: w19 -> [w138]
    tunnel: w18 -> [w128]
    tunnel: w17 -> [w137]
    tunnel: w16 -> [w133]
    tunnel: w15 -> [w130]
    tunnel: w14 -> [w127]
    tunnel: w13 -> [w126]
    tunnel: w12 -> [w123]
    tunnel: w11 -> [w122]
    tunnel: w10 -> [w121]
    tunnel: w9 -> [w120]
    tunnel: w8 -> [w119]
    tunnel: w7 -> [w118]
    tunnel: [w116] -> w6
    tunnel: w5 -> [w116]
    tunnel: [w113] -> w4
    tunnel: w3 -> [w113]
    tunnel: w2 -> [w107]
    tunnel: [w106] -> w1
    tunnel: w28 -> [_]
    tunnel: w27 -> [w174]
    tunnel: w26 -> [w173]
    tunnel: w25 -> [w172]
    tunnel: w24 -> [_]
    tunnel: w6 -> [w171]
    tunnel: w4 -> [w170]
    tunnel: w1 -> [w169]
    frame #0 {
      w35 = T10 4 items=["Grayscale (U8)", "Grayscale (I16)", "Grayscale (SGL)", "Complex (CSG)", "RGB (U32)", "HSL (U32)", "RGB (U64)", "Grayscale (U16)"] ("Image Type")
      w61 = 0.0 ("element")
      w36 = T10 0 items=["Grayscale (U8)", "Grayscale (I16)", "Grayscale (SGL)", "Complex (CSG)", "RGB (U32)", "HSL (U32)", "RGB (U64)", "Grayscale (U16)"] ("Image Type")
      # "Controls definition"
      n2 = case shown="\"16bits\", Default" "bit depth" {
        tunnel: [w103 w105] -> w44
        tunnel: [TRUE FALSE] -> w50
        frame "16bits", Default {
          w103 = T10 7 items=["Grayscale (U8)", "Grayscale (I16)", "Grayscale (SGL)", "Complex (CSG)", "RGB (U32)", "HSL (U32)", "RGB (U64)", "Grayscale (U16)"] ("Image Type")
        }
        frame "8bits" {
          w105 = T10 0 items=["Grayscale (U8)", "Grayscale (I16)", "Grayscale (SGL)", "Complex (CSG)", "RGB (U32)", "HSL (U32)", "RGB (U64)", "Grayscale (U16)"] ("Image Type")
        }
      }
      n3 = Current VI's Path() -> (path=w93:path)
      n4 = Strip Path(path=w93) -> (stripped path=→"path":path)  [unwired: 1 out]
      n5 = call "IMAQ Create"("Image Name"="CCD Image", "Image Type"=w44) -> ("New Image"=w48:T3)  [unwired: 3 in, 1 out]
      n6 = call "IMAQ Create"("Image Name"="CGHy", "Image Type"=w36) -> ("New Image"=w96:T3, "error out"=w95:errorcluster)  [unwired: 3 in]
      n7 = call "IMAQ Create"("Image Name"="Beam X", "Image Type"=w35) -> ("New Image"=w34:T3)  [unwired: 3 in, 1 out]
      n8 = call "IMAQ Create"("Image Name"="CGHx", "Image Type"=w36) -> ("New Image"=w97:T3, "error out"=w94:errorcluster)  [unwired: 3 in]
      n9 = Bundle("2_Xoffset"="2_Xoffset", "2_Yoffset"="2_Yoffset", "2_Xgros"="2_Xgros", "2_Ygros"="2_Ygros", "2_Xfine"="2_Xfine", "2_Yfine"="2_Yfine") -> (w84:T11)  [unwired: 1 in]
      n10 = call "initialize.vi"("14bits"=w50) -> ("session out"=w63:refnum<k35>, "available cameras"=w65:cluster{string[], string[]}, "error out"=w64:errorcluster)  [unwired: 3 in]
      "available\ncameras" <- w65
      n11 = Bundle("1_Xoffset"="1_Xoffset", "1_Yoffset"="1_Yoffset", "1_Xgros"="1_Xgros", "1_Ygros"="1_Ygros", "1_Xfine"="1_Xfine", "1_Yfine"="1_Yfine") -> (w77:T5)  [unwired: 1 in]
      n12 = call "IMAQ Create"("Image Name"="Ref Image", "Image Type"=w44) -> ("New Image"=w46:T3)  [unwired: 3 in, 1 out]
      n13 = call "IMAQ Create"("Image Name"="ROI image", "Image Type"=w44) -> ("New Image"=w43:T3)  [unwired: 3 in, 1 out]
      n14 = Unbundle(w65) -> (w39:string[])  [unwired: 1 out]
      n15 = Array Size(array=w39) -> (size(s)=w60:i32)
      n16 = property on="Camera ID" class="Ring (strict)"("Strings []"=w39) -> ("Value"=w41:u16)  [unwired: 2 in, 2 out]
      n17 = Initialize Array(w61, w60) -> (w62:dbl[])
      n18 = Initialize Array(w61, w60) -> (w59:dbl[])
      n19 = Bundle("1_Radio"="1_Radio", "1_Trans"="1_Trans", "1_Phase"="1_Phase", "1_HoloCode"="1_HoloCode", "1_Semi"="1_Semi", "1_Active"="1_Active", "1_ModType"="1_ModType", "1_Flip"="1_Flip", "HoloNum"="HoloNum", "paramStr"="paramStr", "paramVal"="paramVal", "paramAux"="paramAux") -> (w68:T6)  [unwired: 1 in]
      n20 = Index Array(array=w39, index=0) -> (element=w40:string)
      n21 = case shown="\"Any\", Default" w40 {
        tunnel: [w100 -1 ("Value")] -> w42
        tunnel: w41 -> [w100 _]
        frame "Any", Default {
        }
        frame "NotFound" {
        }
      }
    }
    frame #1 {
      w144 = 1 ("Display")
      # "CHANGE THIS!"
      # "Indicators (setting up)"
      n22 = call "labHolo_path.vi"("sub folder or file (str)"="SupportFiles\\TestPatterns\\no_image.png") -> ("labHolo path"=w108:path)  [unwired: 1 in, 1 out]
      n23 = call "start.vi"("FPS"=w126, "error in (no error)"=w138, "Exposure (ms)"=w127, "Cam id"=w128, "session in"=w137) -> ("error out"=w136:errorcluster, "return value"=w135:T4, "session out"=w134:refnum<k35>)  [unwired: 2 in]
      "camera attr" <- w135
      n24 = call "getSavePath.vi"("beam_name"=w123, "Polarizer"=w122, "Analyzer"=w121, "prefix"=w119, "suffix"=w120) -> ("appended path"=→"defaultPath":string)  [unwired: 10 in]
      n25 = call "positionManager.vi"("Display"=2, "Cluster"=w168) -> ("Y position out"=→"2_Ypos":dbl, "X position out"=→"2_Xpos":dbl)  [unwired: 5 in, 1 out]
      n26 = call "getCalibrationLabels.vi"() -> ("size(s)"=w109:i32, "filenames"=w110:string[])  [unwired: 10 in]
      n27 = Unbundle By Name(w135) -> ("x"=w142:i32, "y"=w141:i32, "FPS"=w125:dbl, "Exposure"=w131:dbl)
      n28 = call "transAndPhaseManager.vi"("Trans in"=w151, "Phase in"=w150) -> ("Trans %"=→"1_T%":dbl, "Intensity"=→"1_Int":dbl, "T gl"=→"1_Tgl":dbl, "Phase Deg"=→"1_PhDeg":dbl, "Phase Rad"=→"1_PhRad":dbl)  [unwired: 9 in]
      n29 = call "positionManager.vi"("Display"=w144, "Cluster"=w159) -> ("Y position out"=→"1_Ypos":dbl, "X position out"=→"1_Xpos":dbl)  [unwired: 5 in, 1 out]
      n30 = call "holoPathEditor.vi"("Display"=w144, "prev. Path"=w108, "input cluster"=w149) -> ("active?"=w112:bool, "appended path"=w111:path)  [unwired: 5 in, 2 out]
      "SLM2 path" <- w111
      "SLM1 path" <- w111
      n31 = call "IMAQ ReadFile"("File Path"=w111, "error in (no error)"=w164, "Image"=w165) -> ("error out"=w163:errorcluster, "Image Out"=w147:T3)  [unwired: 4 in, 3 out]
      n32 = local write "take reff"(FALSE ("take reff")) -> ()
      n33 = property on="SLM calibration" class="Ring (strict)"("Strings []"=w110, "Value"=w109) -> ()  [unwired: 2 in, 2 out]
      n34 = Bundle("x"=w142, "y"=w141) -> (→"image_size":cluster{"x":i32, "y":i32})  [unwired: 1 in]
      n35 = call "IMAQ ReadFile"("File Path"=w108, "Image"=w118) -> ("Image Out"=w117:T3)  [unwired: 5 in, 4 out]
      n36 = call "IMAQ ReadFile"("File Path"=w108, "Image"=w107) -> ("Image Out"=w106:T3)  [unwired: 5 in, 4 out]
      "Beam1" <- w106
      n37 = call "IMAQ ReadFile"("File Path"=w111, "error in (no error)"=w161, "Image"=w162) -> ("error out"=w160:errorcluster, "Image Out"=→"SLM2 monitor" →"CGH_2":T3)  [unwired: 4 in, 3 out]
      n38 = local write "FPS"(w125) -> ()
      n39 = local write "Exposure (ms)"(w131) -> ()
      n40 = Replace Array Subset(array=w133, new element=w131, index=w128) -> (→"exposures":dbl[])
      n41 = Replace Array Subset(array=w130, new element=w125, index=w128) -> (→"FPSs":dbl[])
      n42 = call "showHolo.vi"("Window Number (0...15)"=1, "active?"=w112, "Image"=w147) -> ("Image Out (duplicate)"=→"CGH_1" →"SLM1 monitor":T3)  [unwired: 7 in, 1 out]
      "SLM1 cluster" <- w149
      "1_posCluster" <- w159
      "Reff alert" <- FALSE ("Boolean")
    }
    frame #2 {
      n43 = while {
        shift-right: [w184] -> _
        shift-left: _ -> [w183]
        tunnel: w174 -> [w181]
        tunnel: w173 -> [w180]
        tunnel: w172 -> [w179]
        tunnel: w171 -> [w177]
        tunnel: w170 -> [w176]
        tunnel: w169 -> [w175]
        stop <- w185 stop-if-true
        n44 = event shown="[0] Timeout" {
          selector: _ -> [_ _ _ _ _ _ _ _]
          dyn-events: _ -> [_ _ _ _ _ _ _ _]
          timeout: 1 -> [_ _ _ _ _ _ _ _]
          tunnel: [_ _ _ _ _ _ _ w431] -> w185
          tunnel: [w211 _ _ _ _ _ _ _] -> w184
          tunnel: w183 -> [w222 _ _ _ _ _ _ _]
          tunnel: w181 -> [w220 _ w232 _ _ _ _ _]
          tunnel: w180 -> [w219 _ w231 w264 _ w299 _ _]
          tunnel: w179 -> [w218 _ _ w262 _ _ _ _]
          tunnel: [w217 _ _ w261 _ _ _ _] -> w178
          tunnel: w177 -> [w200 _ _ _ _ _ _ _]
          tunnel: w176 -> [w197 _ _ _ _ _ _ _]
          tunnel: w175 -> [_ _ _ _ _ w295 _ _]
          event Timeout {
            n45 = event-data() -> ()  [unwired: 1 in, 3 out]
            n46 = local read "Camera ID"() -> (w216:u16)
            n47 = call "capture.vi"("error in (no error)"=w218, "Cam ID"=w216, "Image in"=w220, "session in"=w219) -> ("error out"=w217:errorcluster, "Image out"=w201:T3)  [unwired: 3 in, 1 out]
            n48 = local read "bit depth"() -> (w198:enum16{"16bits", "14bits", "12bits", "8bits"})
            n49 = property on="CCD Image" class="ImageControl"() -> ("ROI"=w199:T1)  [unwired: 2 in, 2 out]
            "ROI" <- w199
            n50 = call "histogram.vi"("Image ROI"=w197, "useROI"="Whole/ROI", "ROI Descriptor"=w199, "bit depth"=w198, "Image"=w201) -> ("Statistics"=w207:T12, "Histograph"=→"Histograph":T2, "bins"=w202:i32)  [unwired: 2 in, 2 out]
            n51 = control-ref of="Histograph"() -> (w203:refnum<vi>)
            n52 = Unbundle By Name(w207) -> ("mean (ROI)"=→"mean bar" →"mean":dbl, "max (ROI)"=→"max":i16, "max_counts"=w204:dbl, "image_size"=→"ROI size":i32, "# Sat. Pixels"=→"# Sat. Pixels":sgl)
            n53 = call "setHistogram.vi"("Auto. In"="Auto. hist", "max counts"=w204, "bins"=w202, "WaveformGraph in"=w203) -> ()  [unwired: 7 in, 1 out]
            n54 = local read "RefTimeSeries"() -> (w210:dbl[])
            n55 = local read "RefTimeSeries 2"() -> (w192:dbl[])
            n56 = control-ref of="Reff ROI"() -> (w208:refnum<vi>)
            n57 = Tick Count (ms)() -> (millisecond timer value=w211:u32)
            n58 = call "drawRoi.vi"("bit depth"=w198, "ROI"=w208, "Reff image"=w200, "Whole image"=w201) -> ("size"=→"size":i32, "mean"=w195:dbl, "Image Out"=→"CCD Image":T3, "Percentile alert"=w196:bool)  [unwired: 3 in, 1 out]
            n59 = Subtract(x=w211, y=w222) -> (x-y=w225:u32)
            n60 = Reciprocal(x=w225) -> (1/x=w224:dbl)
            n61 = Insert Into Array(array=w210, new element=w195) -> (w189:dbl[])  [unwired: 1 in]
            n62 = property on="Reff alert" class="Bool (strict)"("Blinking"=w196) -> ()  [unwired: 2 in, 2 out]
            n63 = call <vilib>:"Std Deviation and Variance.vi"("X"=w189) -> ("mean"=w188:dbl, "standard deviation"=w187:dbl)  [unwired: 1 in, 1 out]
            n64 = Multiply(x=u32 1000 ("y"), y=w224) -> (x*y=→"Real FPS":dbl)
            n65 = local write "RefTimeSeries"(w189) -> ()
            n66 = Add(x=w188, y=w187) -> (x+y=w186:dbl)
            n67 = Insert Into Array(array=w192, new element=w186) -> (w190:dbl[])  [unwired: 1 in]
            n68 = Build Array(w189, w190) -> (→"Chart TimeSeries":dbl[][])
            n69 = local write "RefTimeSeries 2"(w190) -> ()
          }
          event "take reff", "Reset reff.": Value Change {
            w229 = dbl[] [] ("RefTimeSeries")
            w228 = FALSE ("take reff")
            n70 = event-data() -> ("CtlRef"=w227:refnum<vi>)  [unwired: 1 in, 5 out]
            n71 = property class="Bool (strict)"(reference=w227) -> ("Label.Text"=w226:string)  [unwired: 1 in, 2 out]
            n72 = case shown="\"Any\", Default" w226 {
              frame "Any", Default {
              }
              frame "take reff" {
                n73 = property on="CCD Image" class="ImageControl"() -> ("ROI"=→"Reff ROI":T1)  [unwired: 2 in, 2 out]
              }
            }
            n74 = local write "Reset reff."(w228) -> ()
            n75 = local write "take reff"(w228) -> ()
            n76 = local write "RefTimeSeries 2"(w229) -> ()
            n77 = local write "RefTimeSeries"(w229) -> ()
          }
          event "suffix", "Polarizer", "Analyzer", "beam_name", "Save": Value Change {
            n78 = event-data() -> ("CtlRef"=w235:refnum<vi>)  [unwired: 1 in, 5 out]
            n79 = local read "beam_name"() -> (w240:string)
            n80 = property class="Ctl"(reference=w235) -> ("Label.Text"=w234:string)  [unwired: 1 in, 2 out]
            n81 = local read "paramAux"() -> (w237:string)
            n82 = local read "Polarizer"() -> (w239:string)
            n83 = local read "Analyzer"() -> (w238:string)
            n84 = local read "suffix"() -> (w236:string)
            n85 = call "getSavePath.vi"("beam_name"=w240, "Polarizer"=w239, "Analyzer"=w238, "prefix"=w237, "suffix"=w236) -> ("appended path"=w233:string)  [unwired: 10 in]
            n86 = case shown="\"Save\"" w234 {
              tunnel: w233 -> [_ w243]
              tunnel: w232 -> [_ w242]
              tunnel: w231 -> [_ w241]
              frame "Any", Default {
              }
              frame "Save" {
                n87 = stacked-sequence {
                  tunnel: [_ w253 _] -> _
                  tunnel: w243 -> [_ w252 _]
                  tunnel: w242 -> [_ w251 _]
                  tunnel: w241 -> [_ w246 _]
                  frame #0 {
                    n88 = property on="Save" class="Bool (strict)"("DisabledEnum"=T9."Disabled and Grayed Out" ("Disabled")) -> ()  [unwired: 2 in, 2 out]
                  }
                  frame #1 {
                    n89 = local read "Reff ROI"() -> (w250:T1)
                    n90 = local read "bit depth"() -> (w245:enum16{"16bits", "14bits", "12bits", "8bits"})
                    n91 = property on="CCD Image" class="ImageControl"() -> ("ROI"=w249:T1)  [unwired: 2 in, 2 out]
                    n92 = Unbundle By Name(w249) -> ("Global Rectangle"=w248:i32[])
                    n93 = Unbundle By Name(w250) -> ("Global Rectangle"=w247:i32[])
                    n94 = call "saveImage.vi"("bit depth"=w245, "session in"=w246, "reff ROI"=w247, "main ROI"=w248, "appended path"=w252, "Refnum in"=w251) -> ("error out"=w253:errorcluster)  [unwired: 4 in, 1 out]
                  }
                  frame #2 {
                    n95 = property on="Save" class="Bool (strict)"("DisabledEnum"=T9."Enabled" ("Disabled"), "Value"=FALSE ("Save")) -> ()  [unwired: 2 in, 2 out]
                  }
                }
              }
            }
            n96 = local write "defaultPath"(w233) -> ()
          }
          event "FPS", "Exposure (ms)": Value Change {
            n97 = event-data() -> ("CtlRef"=w258:refnum<vi>, "NewVal"=w263:dbl)  [unwired: 1 in, 4 out]
            n98 = property class="DigNum (strict)"(reference=w258) -> ("Label.Text"=w259:string)  [unwired: 1 in, 2 out]
            n99 = local read "Camera ID"() -> (w260:u16)
            n100 = case shown="\"Exposure (ms)\", Default" w259 {
              tunnel: w264 -> [w270 w277]
              tunnel: w263 -> [w269 w276]
              tunnel: w262 -> [w268 w275]
              tunnel: [w267 w274] -> w261
              tunnel: w260 -> [_ w273]
              tunnel: [w265 w272] -> w256
              tunnel: [w266 w271] -> w257
              frame "Exposure (ms)", Default {
                n101 = call "set_exposure.vi"("error in (no error)"=w268, "exposure"=w269, "Session in"=w270) -> ("error out"=w267:errorcluster, "true FPS"=w265:dbl, "true exposure"=w266:dbl)  [unwired: 4 in, 1 out]
              }
              frame "FPS" {
                n102 = call "set_fps.vi"("error in (no error)"=w275, "cam ID"=w273, "FPS"=w276, "Session in"=w277) -> ("error out"=w274:errorcluster, "true Exposure"=w271:dbl, "true FPS"=w272:dbl)  [unwired: 3 in, 1 out]
              }
            }
            n103 = local write "Exposure (ms)"(w257) -> ()
            n104 = local write "FPS"(w256) -> ()
          }
          event "Camera ID": Value Change {
            n105 = event-data() -> ("OldVal"=w279:u16, "NewVal"=w278:u16)  [unwired: 1 in, 4 out]
            n106 = flat-sequence {
              tunnel: w279 -> [w286]
              tunnel: w278 -> [w291]
              frame #0 {
                n107 = local read "exposures"() -> (w284:dbl[])
                n108 = local read "Exposure (ms)"() -> (w285:dbl)
                n109 = local read "FPSs"() -> (w281:dbl[])
                n110 = local read "FPS"() -> (w282:dbl)
                n111 = Replace Array Subset(array=w281, new element=w282, index=w286) -> (w280:dbl[])
                n112 = Replace Array Subset(array=w284, new element=w285, index=w286) -> (w283:dbl[])
                n113 = local write "FPSs"(w280) -> ()
                n114 = local write "exposures"(w283) -> ()
              }
              frame #1 {
                n115 = local read "FPSs"() -> (w289:dbl[])
                n116 = local read "exposures"() -> (w290:dbl[])
                n117 = Index Array(array=w290, index=w291) -> (element=w288:dbl)
                n118 = Index Array(array=w289, index=w291) -> (element=w287:dbl)
                n119 = local write "FPS"(w287) -> ()
                n120 = local write "Exposure (ms)"(w288) -> ()
              }
            }
          }
          event "1_Radio", "1_Trans", "HoloNum", "1_ModType", "1_Semi", "1_Active", "paramVal", "paramStr", "paramAux", "1_Phase", "1_Flip": Value Change {
            w296 = 1 ("Display")
            # "Old"
            # "New"
            # "SLM number (display)"
            n121 = event-data() -> ("CtlRef"=w316:refnum<vi>, "OldVal"=w320:variant, "NewVal"=w303:variant)  [unwired: 1 in, 3 out]
            n122 = local read "SLM1 cluster"() -> (w318:T6)
            n123 = local read "SLM1 path"() -> (w297:path)
            n124 = call "updateHoloBundle.vi"("NewValue"=w303, "input cluster"=w318, "CtlRef"=w316) -> ("output cluster"=w298:T13)  [unwired: 7 in, 1 out]
            n125 = property class="Ctl"(reference=w316) -> ("Label.Text"=w317:string)  [unwired: 1 in, 2 out]
            n126 = local read "CGH_1"() -> (w319:T3)
            n127 = call "getHologram.vi"("Display"=w296, "session in"=w299, "previous path"=w297, "options cluster"=w298, "Beam in"=w295, "Hologram in"=w319) -> ("error out"=→"path editor log":errorcluster, "appended path"=w292:path, "Beam out"=w294:T3, "Hologram out"=w300:T3, "file or folder exists?"=w293:bool)  [unwired: 1 in]
            n128 = case shown="\"ParamVal\"" w317 {
              tunnel: w320 -> [w322 w328 _ w334 _ w345 w351 w357 _ _]
              tunnel: w303 -> [_ _ _ _ w343 _ _ _ w366 w370]
              tunnel: w292 -> [_ _ _ _ _ _ _ _ _ _]
              tunnel: w293 -> [w321 w327 _ w333 _ w344 w350 w356 _ _]
              frame "HoloNum" {
                n129 = case shown="False" w321 {
                  tunnel: w322 -> [w323 _]
                  frame False {
                    n130 = feedback #1() -> (w324:dbl)  [unwired: 1 in]
                    n131 = Variant To Data(type=w324, Variant=w323) -> (data=w326:dbl)  [unwired: 1 in, 1 out]
                    n132 = property on="HoloNum" class="DigNum (strict)"("Value"=w326) -> ("Value"=w325:dbl)  [unwired: 2 in, 2 out]
                    n133 = feedback-in #1(w325) -> ()
                  }
                  frame True {
                  }
                }
              }
              frame "ParamStr" {
                n134 = case shown="False" w327 {
                  tunnel: w328 -> [w329 _]
                  frame False {
                    n135 = feedback #2() -> (w330:string)  [unwired: 1 in]
                    n136 = Variant To Data(type=w330, Variant=w329) -> (data=w332:string)  [unwired: 1 in, 1 out]
                    n137 = property on="paramStr" class="Str"("Value"=w332) -> ("Value"=w331:string)  [unwired: 2 in, 2 out]
                    n138 = feedback-in #2(w331) -> ()
                  }
                  frame True {
                  }
                }
              }
              frame "Any", Default {
              }
              frame "ParamVal" {
                n139 = case shown="False" w333 {
                  tunnel: w334 -> [w335 _]
                  frame False {
                    n140 = feedback #3() -> (w336:i64)  [unwired: 1 in]
                    n141 = Variant To Data(type=w336, Variant=w335) -> (data=w338:i64)  [unwired: 1 in, 1 out]
                    n142 = property on="paramVal" class="DigNum (strict)"("Value"=w338) -> ("Value"=w337:i64)  [unwired: 2 in, 2 out]
                    n143 = feedback-in #3(w337) -> ()
                  }
                  frame True {
                  }
                }
              }
              frame "1_Active" {
                n144 = Variant To Data(type=0, Variant=w343) -> (data=w339:i32)  [unwired: 1 in, 1 out]
                n145 = Not Equal?(x=u16 0, y=w339) -> (x != y?=w340:bool)
                n146 = property on="1_Active" class="Ring (strict)"("Blinking"=w340) -> ()  [unwired: 2 in, 2 out]
              }
              frame "ParamAux" {
                n147 = case shown="False" w344 {
                  tunnel: w345 -> [w346 _]
                  frame False {
                    n148 = feedback #4() -> (w347:string)  [unwired: 1 in]
                    n149 = Variant To Data(type=w347, Variant=w346) -> (data=w349:string)  [unwired: 1 in, 1 out]
                    n150 = property on="paramAux" class="Str"("Value"=w349) -> ("Value"=w348:string)  [unwired: 2 in, 2 out]
                    n151 = feedback-in #4(w348) -> ()
                  }
                  frame True {
                  }
                }
              }
              frame "1_ModType" {
                n152 = case shown="False" w350 {
                  tunnel: w351 -> [w352 _]
                  frame False {
                    n153 = feedback #5() -> (w355:string)  [unwired: 1 in]
                    n154 = Variant To Data(type=w355, Variant=w352) -> (data=w353:string)  [unwired: 1 in, 1 out]
                    n155 = property on="1_ModType" class="CmbBox"("Value"=w353) -> ("Value"=w354:string)  [unwired: 2 in, 2 out]
                    n156 = feedback-in #5(w354) -> ()
                  }
                  frame True {
                  }
                }
              }
              frame "1_Radio" {
                n157 = case shown="False" w356 {
                  tunnel: w357 -> [w360 _]
                  frame False {
                    n158 = Variant To Data(type=0, Variant=w360) -> (data=w358:i32)  [unwired: 1 in, 1 out]
                    n159 = local write "1_Radio"(w358) -> ()
                  }
                  frame True {
                  }
                }
              }
              frame "1_Trans" {
                n160 = Variant To Data(type=0.0, Variant=w366) -> (data=w364:dbl)  [unwired: 1 in, 1 out]
                n161 = call "transAndPhaseManager.vi"("Trans in"=w364) -> ("Trans %"=w363:dbl, "Intensity"=w362:dbl, "T gl"=w361:dbl)  [unwired: 10 in, 2 out]
                n162 = local write "1_T%"(w363) -> ()
                n163 = local write "1_Int"(w362) -> ()
                n164 = local write "1_Tgl"(w361) -> ()
              }
              frame "1_Phase" {
                n165 = Variant To Data(type=0.0, Variant=w370) -> (data=w367:dbl)  [unwired: 1 in, 1 out]
                n166 = call "transAndPhaseManager.vi"("Phase in"=w367) -> ("Phase Deg"=w369:dbl, "Phase Rad"=w368:dbl)  [unwired: 10 in, 3 out]
                n167 = local write "1_PhDeg"(w369) -> ()
                n168 = local write "1_PhRad"(w368) -> ()
              }
            }
            n169 = local write "SLM1 cluster"(w298) -> ()
            n170 = local write "SLM1 path"(w292) -> ()
            n171 = local write "Beam1"(w294) -> ()
            n172 = local read "1_Active"() -> (w304:u16)
            n173 = local read "1_Radio"() -> (w305:T8)
            n174 = local write "SLM1 monitor"(w300) -> ()
            n175 = local write "CGH_1"(w300) -> ()
            n176 = case shown="0" w304 {
              tunnel: [w374 w388 w402] -> w306
              tunnel: [w374 T9."Enabled" ("Disabled") w402] -> w309
              tunnel: [w374 w387 w402] -> w307
              tunnel: [w374 w386 w402] -> w310
              tunnel: [w374 w385 w402] -> w311
              tunnel: [w374 w384 w402] -> w308
              tunnel: [w374 w382 w402] -> w312
              tunnel: [w374 w381 w402] -> w313
              tunnel: [w374 w380 w402] -> w314
              tunnel: [w374 w379 w402] -> w315
              tunnel: w305 -> [_ w378 _]
              tunnel: [w374 T9."Enabled" ("Disabled") w402] -> w302
              tunnel: w296 -> [w373 w375 w401]
              tunnel: w300 -> [_ w376 w400]
              frame 1, Default {
                w374 = T9."Disabled and Grayed Out" ("Disabled")
                # "Hide CGH windows"
                # "OFF"
                n177 = call "IMAQ WindShow"("Hide/Show (Show)"=FALSE, "Window Number (0...15)"=w373) -> ()  [unwired: 4 in, 3 out]
              }
              frame 0 {
                # "ON"
                n178 = case shown="\"Radio Selection 8\"" w378 {
                  tunnel: [w389 w390 w392 w395 w396 w399] -> w388
                  tunnel: [w389 T9."Enabled" ("Disabled") w392 w394 w397 w399] -> w387
                  tunnel: [w389 w390 w393 w395 w397 w398] -> w386
                  tunnel: [w389 w390 w392 w395 w397 w398] -> w385
                  tunnel: [w389 w390 w393 w395 w397 w398] -> w384
                  tunnel: [w389 w390 w392 w394 w396 w398] -> w382
                  tunnel: [w389 w390 w392 w394 w396 w398] -> w381
                  tunnel: [w389 w390 w392 w394 w396 w398] -> w380
                  tunnel: [w389 w390 w392 w394 w396 w398] -> w379
                  frame "Radio Selection 1", Default {
                    w389 = T9."Disabled and Grayed Out" ("Disabled")
                    # "Browser holo\n(Default)"
                  }
                  frame "Radio Selection 3" {
                    w390 = T9."Disabled and Grayed Out" ("Disabled")
                  }
                  frame "Radio Selection 4" {
                    w393 = T9."Enabled" ("Disabled")
                    w392 = T9."Disabled and Grayed Out" ("Disabled")
                    # "Gray level"
                  }
                  frame "Radio Selection 5" {
                    w394 = T9."Enabled" ("Disabled")
                    w395 = T9."Disabled and Grayed Out" ("Disabled")
                    # "Hologram prefabricated"
                  }
                  frame "Radio Selection 6" {
                    w396 = T9."Disabled and Grayed Out" ("Disabled")
                    w397 = T9."Enabled" ("Disabled")
                    # "Complex arbitrary value"
                  }
                  frame "Radio Selection 8" {
                    w398 = T9."Disabled and Grayed Out" ("Disabled")
                    w399 = T9."Enabled" ("Disabled")
                    # "code editor"
                  }
                }
                n179 = call "showHolo.vi"("Window Number (0...15)"=w375, "Image"=w376) -> ()  [unwired: 8 in, 2 out]
              }
              frame 2 {
                w402 = T9."Enabled" ("Disabled")
                # "edit"
                n180 = call "showHolo.vi"("Window Number (0...15)"=w401, "Image"=w400) -> ()  [unwired: 8 in, 2 out]
                n181 = property on="1_Active" class="Ring (strict)"("Blinking"=FALSE) -> ()  [unwired: 2 in, 2 out]
              }
            }
            n182 = property on="1_Xoffset" class="DigNum (strict)"("DisabledEnum"=w302) -> ()  [unwired: 2 in, 2 out]
            n183 = property on="HoloNum" class="DigNum (strict)"("DisabledEnum"=w312) -> ()  [unwired: 2 in, 2 out]
            n184 = property on="1_Yoffset" class="DigNum (strict)"("DisabledEnum"=w302) -> ()  [unwired: 2 in, 2 out]
            n185 = property on="paramStr" class="Str"("DisabledEnum"=w313) -> ()  [unwired: 2 in, 2 out]
            n186 = property on="1_Xgros" class="Slide (strict)"("DisabledEnum"=w302) -> ()  [unwired: 2 in, 2 out]
            n187 = property on="paramVal" class="DigNum (strict)"("DisabledEnum"=w314) -> ()  [unwired: 2 in, 2 out]
            n188 = property on="1_Ygros" class="Slide (strict)"("DisabledEnum"=w302) -> ()  [unwired: 2 in, 2 out]
            n189 = property on="1_ModType" class="CmbBox"("DisabledEnum"=w307) -> ()  [unwired: 2 in, 2 out]
            n190 = property on="1_Trans" class="Slide (strict)"("DisabledEnum"=w310) -> ()  [unwired: 2 in, 2 out]
            n191 = property on="1_Phase" class="Slide (strict)"("DisabledEnum"=w311) -> ()  [unwired: 2 in, 2 out]
            n192 = property on="1_Semi" class="Bool (strict)"("DisabledEnum"=w308) -> ()  [unwired: 2 in, 2 out]
            n193 = property on="1_Radio" class="RadioBtnsControl (strict)"("DisabledEnum"=w309) -> ()  [unwired: 2 in, 2 out]
            n194 = property on="1_HoloCode" class="Str"("DisabledEnum"=w306) -> ()  [unwired: 2 in, 2 out]
            n195 = property on="paramAux" class="Str"("DisabledEnum"=w315) -> ()  [unwired: 2 in, 2 out]
            n196 = property on="1_Xfine" class="Slide (strict)"("DisabledEnum"=w302) -> ()  [unwired: 2 in, 2 out]
            n197 = property on="1_Int" class="DigNum (strict)"("DisabledEnum"=w310) -> ()  [unwired: 2 in, 2 out]
            n198 = property on="1_Flip" class="CmbBox"("DisabledEnum"=w309) -> ()  [unwired: 2 in, 2 out]
            n199 = property on="1_PhRad" class="DigNum (strict)"("DisabledEnum"=w311) -> ()  [unwired: 2 in, 2 out]
            n200 = property on="1_T%" class="DigNum (strict)"("DisabledEnum"=w310) -> ()  [unwired: 2 in, 2 out]
            n201 = property on="1_Tgl" class="DigNum (strict)"("DisabledEnum"=w310) -> ()  [unwired: 2 in, 2 out]
            n202 = property on="1_PhDeg" class="DigNum (strict)"("DisabledEnum"=w311) -> ()  [unwired: 2 in, 2 out]
            n203 = property on="1_Yfine" class="Slide (strict)"("DisabledEnum"=w302) -> ()  [unwired: 2 in, 2 out]
          }
          event "1_Xoffset", "1_Yoffset", "1_Xgros", "1_Ygros", "1_Xfine", "1_Yfine": Value Change {
            n204 = event-data() -> ("CtlRef"=w411:refnum<vi>, "NewVal"=w408:dbl)  [unwired: 1 in, 4 out]
            n205 = property class="Num"(reference=w411) -> ("Label.Text"=w410:string)  [unwired: 1 in, 2 out]
            n206 = local read "1_posCluster"() -> (w409:T5)
            n207 = case shown="\"1_Xoffset\"" w410 {
              tunnel: w409 -> [w414 w417 w420 w423 w426 w429 w430]
              tunnel: w408 -> [w413 w416 w419 w422 w425 w428 _]
              tunnel: [w412 w415 w418 w421 w424 w427 w430] -> w407
              frame "1_Xoffset" {
                n208 = Bundle By Name(cluster=w414, "1_Xoffset"=w413) -> (w412:T5)
              }
              frame "1_Yoffset" {
                n209 = Bundle By Name(cluster=w417, "1_Yoffset"=w416) -> (w415:T5)
              }
              frame "1_Xgros" {
                n210 = Bundle By Name(cluster=w420, "1_Xgros"=w419) -> (w418:T5)
              }
              frame "1_Ygros" {
                n211 = Bundle By Name(cluster=w423, "1_Ygros"=w422) -> (w421:T5)
              }
              frame "1_Xfine" {
                n212 = Bundle By Name(cluster=w426, "1_Xfine"=w425) -> (w424:T5)
              }
              frame "1_Yfine" {
                n213 = Bundle By Name(cluster=w429, "1_Yfine"=w428) -> (w427:T5)
              }
              frame "Any", Default {
              }
            }
            n214 = local write "1_posCluster"(w407) -> ()
            n215 = call "positionManager.vi"("Display"=1 ("Window Number (0...15)"), "Cluster"=w407) -> ("Y position out"=w405:dbl, "X position out"=w406:dbl)  [unwired: 5 in, 1 out]
            n216 = local write "1_Xpos"(w406) -> ()
            n217 = local write "1_Ypos"(w405) -> ()
          }
          event "Parada Total": Value Change {
            n218 = event-data() -> ("NewVal"=w431:bool)  [unwired: 1 in, 5 out]
          }
        }
        "py error" <- w178
      }
    }
    frame #3 {
      n219 = property on="Parada Total" class="Bool (strict)"("Value"=FALSE ("Parada Total")) -> ()  [unwired: 2 in, 2 out]
      n220 = call "IMAQ WindClose"("Close All Windows (False)"=TRUE) -> ()  [unwired: 5 in, 1 out]
    }
  }
